vi "SetUTChanEnabSts.vi"(8 "错误输入（无错误）":errorcluster, 10 "使能状态":u8) -> (0 "错误输出":errorcluster)   [LabVIEW 2014]
uses:
  X86Dll/ZXUTConfigMgr.dll
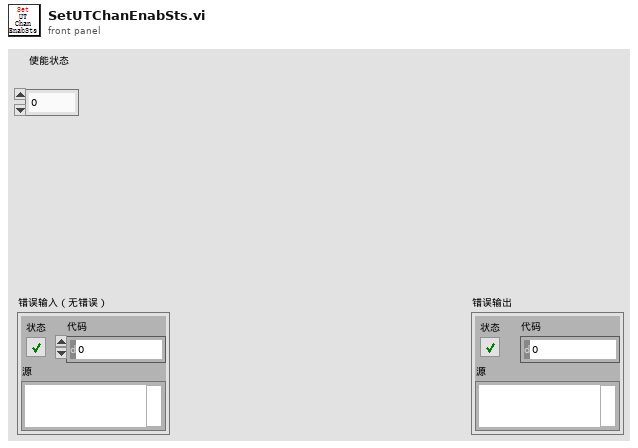
[diagram p1: front panel]
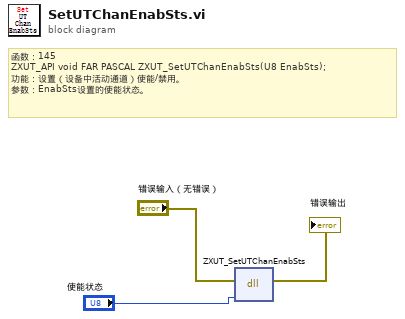
[diagram p0: block diagram]
diagram:
  # "函数：145\nZXUT_API void\tFAR PASCAL ZXUT_SetUTChanEnabSts(U8 EnabSts);\n功能：设置（设备中活动通道）使能/禁用。\n参数：EnabSts设置的使能状态。"
  n1 = dll-call lib="D:/Software/Utrasonic on-line monitoring/X86Dll/ZXUTConfigMgr.dll" fn="ZXUT_SetUTChanEnabSts"(error in="错误输入（无错误）", "EnabSts"="使能状态") -> (error out=→"错误输出":errorcluster)  [unwired: 4 in, 1 out]
